vi "Add Class Documentation.vi"(10 "Class URL Format":string, 11 "Class":refnum<vi>) -> (3 "Class Dup":refnum<vi>)   [LabVIEW 2013]
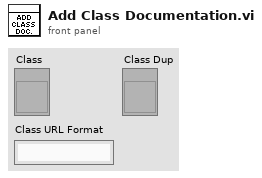
[diagram p1: front panel]
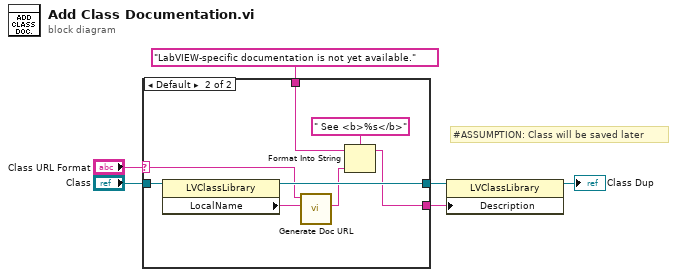
[diagram p0: block diagram]
diagram:
  # "#ASSUMPTION: Class will be saved later"
  n1 = case shown="Default" "Class URL Format" {
    selector: "Class URL Format" -> [_ w9]
    tunnel: "Class" -> [w8 w16]
    tunnel: "LabVIEW-specific documentation is not yet available." -> [w7 w15]
    tunnel: [w8 w13] -> w3
    tunnel: [w7 w11] -> w2
    frame "" {
      # "No URL format specified"
    }
    frame Default {
      n2 = property class="LVClassLibrary"(reference=w16) -> (reference out=w13:refnum<vi>, "LocalName"=w14:string)  [unwired: 1 in, 1 out]
      n3 = call "Generate Doc URL.vi"("Owning Entity Name"=w14, "URL Format"=w9) -> ("Final URL"=w12:string)  [unwired: 9 in]
      n4 = Format Into String(format string=" See <b>%s</b>", initial string=w15, w12) -> (resulting string=w11:string)  [unwired: 1 in, 1 out]
    }
  }
  n5 = property class="LVClassLibrary"(reference=w3, "Description"=w2) -> (reference out=→"Class Dup":refnum<vi>)  [unwired: 1 in, 1 out]
